vi "标识说明.vi"() -> ()   [LabVIEW 2016, in "数据查询.lvlib"]
uses:
  <vilib>/Utility/miscctls.llb/LVPositionTypeDef.ctl
  <vilib>/Utility/miscctls.llb/LVPointTypeDef.ctl
panel:
  in  "标识说明":i32(listbox)
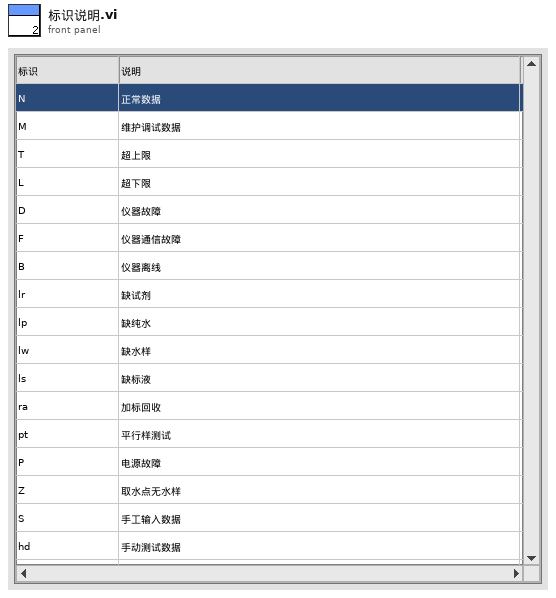
[diagram p1: front panel]
types:
  T1 = typedef "LVPointTypeDef.ctl" = cluster{"Horizontal":i16, "Vertical":i16}
  T2 = typedef "LVPositionTypeDef.ctl" = cluster{"Left":i32, "Top":i32}
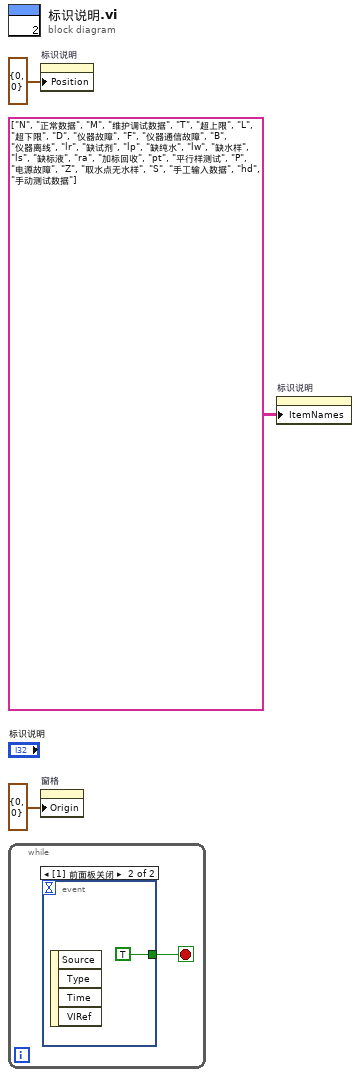
[diagram p0: block diagram]
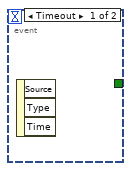
[diagram p2: hidden frame]
diagram:
  n1 = while {
    stop <- w4 stop-if-true
    n2 = event shown="[1] 前面板关闭" {
      selector: _ -> [_ _]
      dyn-events: _ -> [_ _]
      timeout: _ -> [_ _]
      tunnel: [_ TRUE] -> w4
      event Timeout {
        n3 = event-data() -> ()  [unwired: 1 in, 3 out]
      }
      event Panel Close {
        n4 = event-data() -> ()  [unwired: 1 in, 4 out]
      }
    }
  }
  n5 = property on="标识说明" class="MCListbox (严格)"("Position"=T2 {"Left"=0, "Top"=0} ("位置")) -> ()  [unwired: 2 in, 2 out]
  n6 = property on="窗格" class="Pane"("Origin"=T1 {"Horizontal"=0, "Vertical"=0} ("原点")) -> ()  [unwired: 2 in, 2 out]
  n7 = property on="标识说明" class="MCListbox (严格)"("ItemNames"=string[][] [["N", "正常数据"], ["M", "维护调试数据"], ["T", "超上限"], ["L", "超下限"], ["D", "仪器故障"], ["F", "仪器通信故障"], ["B", "仪器离线"], ["lr", "缺试剂"], ["lp", "缺纯水"], ["lw", "缺水样"], ["ls", "缺标液"], ["ra", "加标回收"], ["pt", "平行样测试"], ["P", "电源故障"], ["Z", "取水点无水样"], ["S", "手工输入数据"], ["hd", "手动测试数据"]]) -> ()  [unwired: 2 in, 2 out]
